vi "dllTest-ocr.vi"() -> ()   [LabVIEW 2025]
uses:
  Rectangle.ctl
  TextDecRecResult2L.ctl
panel:
  out "succ 3":i32
  out "succ 2":i32
  out "succ 5":i32
  out "deviceNum":i32
  out "succ":i32
  out "tcv":u64
  out "Image":T1(plugin-control)
  in  "PathImage":path=path "D:/Test/dllTest/images_2"
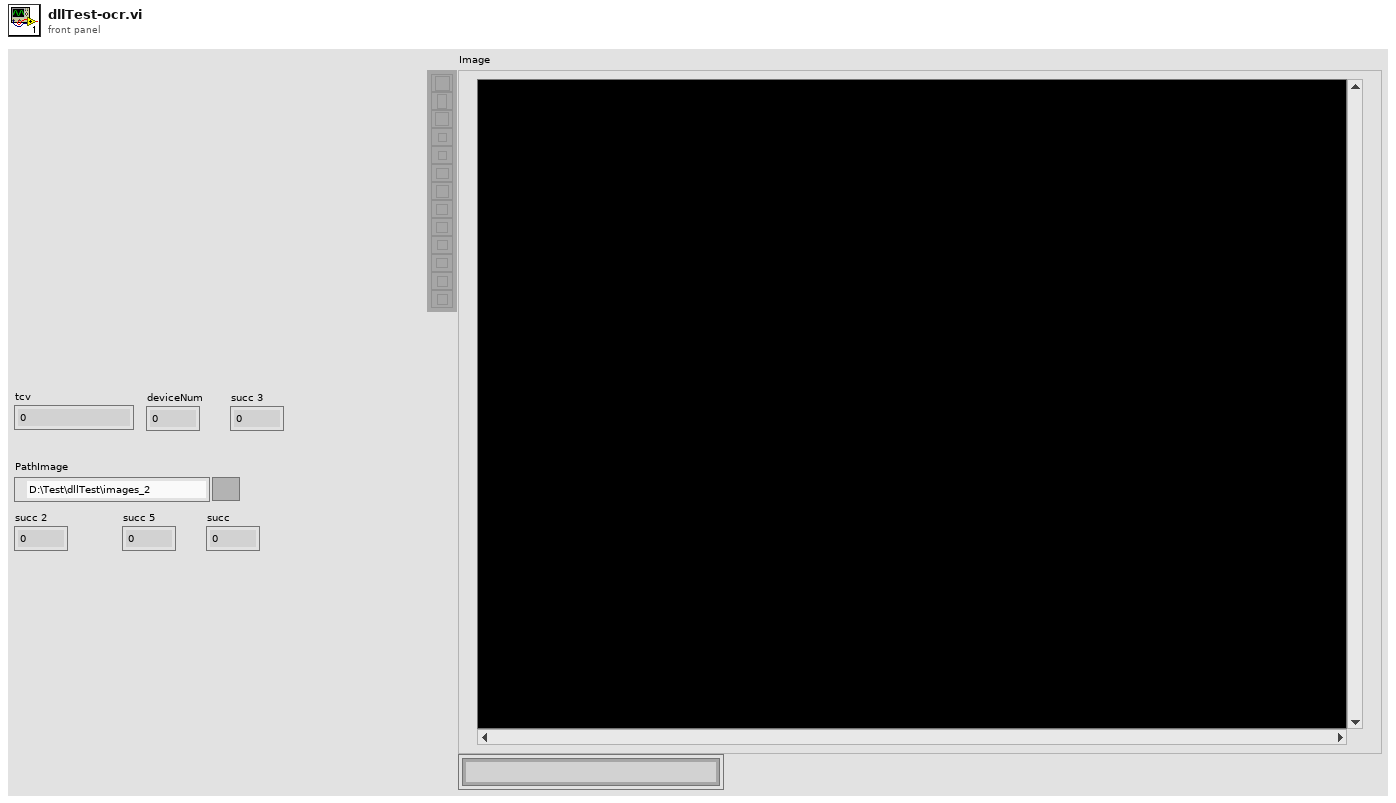
[diagram p1: front panel]
types:
  T1 = typedef "IMAQ Image.ctl" = refnum<image>
  T2 = typedef "Rectangle.ctl" = cluster{"T":i32, "L":i32, "B":i32, "R":i32}
  T3 = typedef "TextDecRecResult2L.ctl" = cluster{"imgIdx":i32, "TLx":i32, "TLy":i32, "BRx":i32, "BRy":i32, "angle":sgl, "txtLen":i32}
  T4 = cluster{"imgIdx":i32, "TLx":i32, "TLy":i32, "BRx":i32, "BRy":i32, "angle":sgl, "txtLen":i32}
  T5 = enum32{"Map Pixel Pointer", "Unmap Pixel Pointer", "Get Pixels Infos"}
  T6 = cluster{"imgIdx":i32, "TLx":i32, "TLy":i32, "BRx":i32, "BRy":i32, "angle":sgl, "txtLen":i32}[]
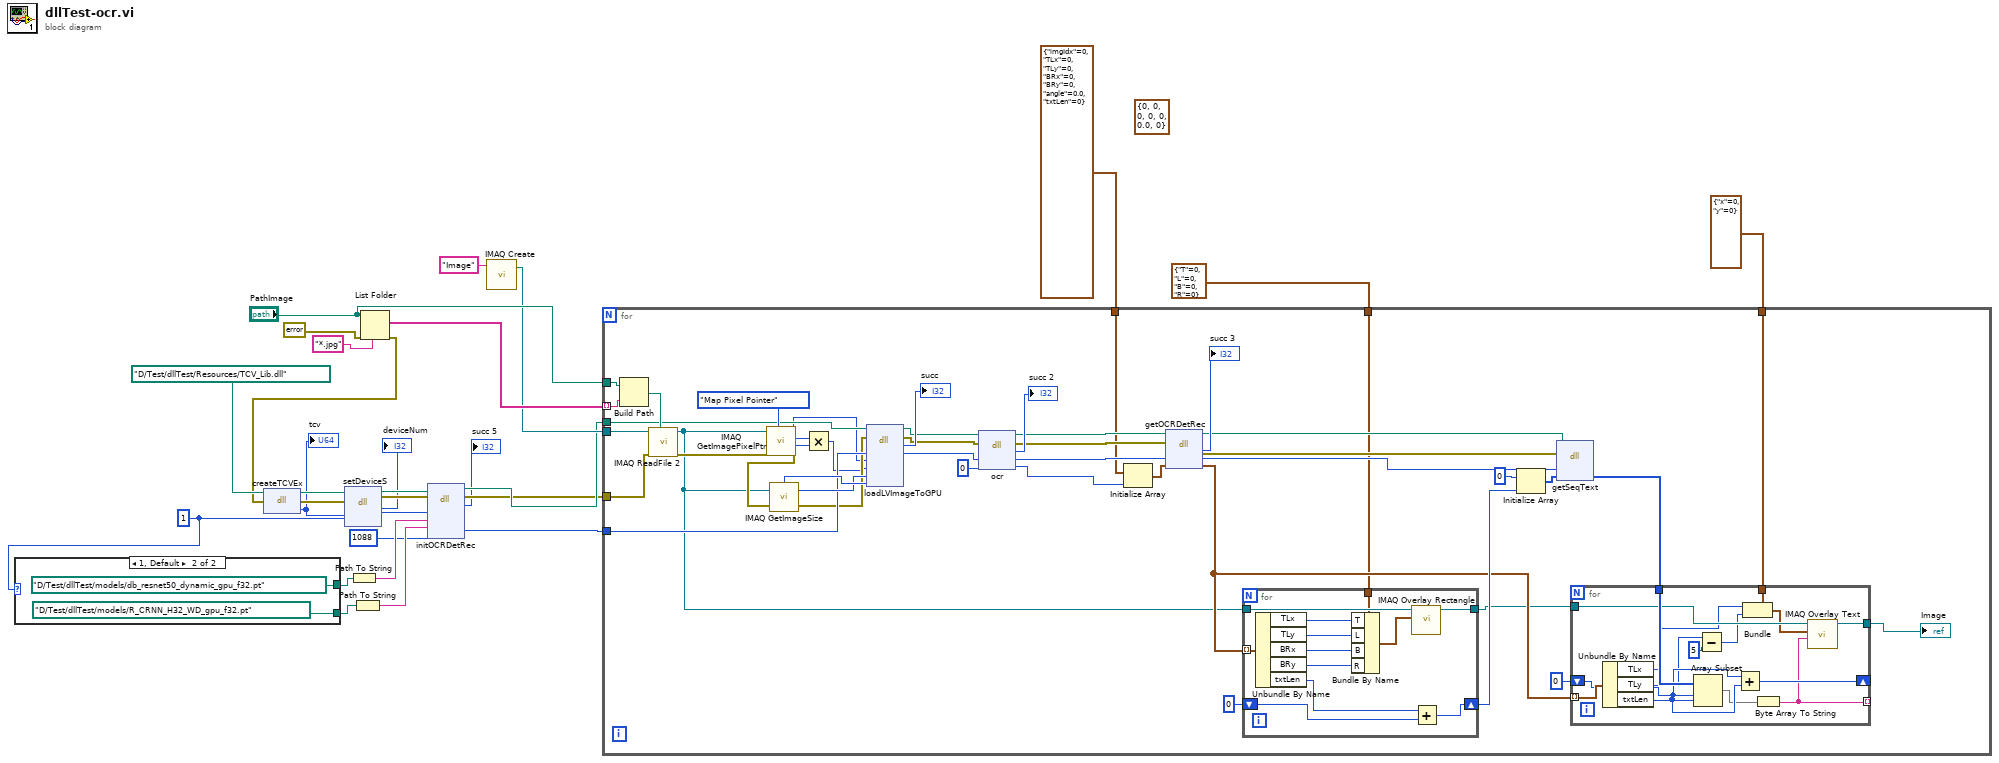
[diagram p0: block diagram]
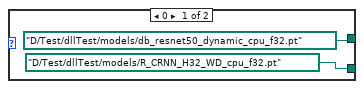
[diagram p2: hidden frame]
diagram:
  (unwired) T3 {"imgIdx"=0, "TLx"=0, "TLy"=0, "BRx"=0, "BRy"=0, "angle"=0.0, "txtLen"=0}
  w3 = 1 ("device")
  n1 = case shown="1, Default" w3 {
    tunnel: [path "D:/Test/dllTest/models/R_CRNN_H32_WD_cpu_f32.pt" ("PathModelR") path "D:/Test/dllTest/models/R_CRNN_H32_WD_gpu_f32.pt" ("PathModelR")] -> w2
    tunnel: [path "D:/Test/dllTest/models/db_resnet50_dynamic_cpu_f32.pt" ("PathModelD") path "D:/Test/dllTest/models/db_resnet50_dynamic_gpu_f32.pt" ("PathModelD")] -> w1
    frame 0 {
    }
    frame 1, Default {
    }
  }
  n2 = Path To String(path=w1) -> (string=w17:string)
  n3 = Path To String(path=w2) -> (string=w16:string)
  n4 = List Folder(path="PathImage", pattern="*.jpg", error in=errorcluster {"status"=FALSE, "code"=0, "source"=""}) -> (filenames=w26:string[], error out=w21:errorcluster)  [unwired: 1 in, 2 out]
  n5 = dll-call lib="D:/Test/dllTest/Resources/TCV_Lib.dll" fn="createTCVEx"(path in=path "D:/Test/dllTest/Resources/TCV_Lib.dll", error in=w21) -> (path out=w15:path, error out=w14:errorcluster, "tcv"=w13:u64)  [unwired: 1 in]
  "tcv" <- w13
  n6 = dll-call lib="D:/Test/dllTest/Resources/TCV_Lib.dll" fn="setDeviceS"(path in=w15, error in=w14, "TCV"=w13, "device"=w3) -> (path out=w12:path, error out=w11:errorcluster, "deviceNum"=→"deviceNum":i32, "TCV"=w10:u64)  [unwired: 2 in]
  n7 = dll-call lib="D:/Test/dllTest/Resources/TCV_Lib.dll" fn="initOCRDetRec"(path in=w12, error in=w11, "TCV"=w10, "modelPathD"=w17, "modelPathD"=w16, "targetSize"=1088) -> (path out=w20:path, error out=w19:errorcluster, "succ"=→"succ 5":i32, "TCV"=w18:u64)  [unwired: 4 in]
  n8 = call "IMAQ Create"("Image Name"="Image") -> ("New Image"=w24:T1)  [unwired: 4 in, 1 out]
  n9 = for {
    tunnel: "PathImage" -> [w77]
    tunnel: w26 -> [w76] mode=indexing
    tunnel: w24 -> [w74]
    tunnel: w18 -> [w69]
    tunnel: w20 -> [w68]
    tunnel: w19 -> [w60]
    tunnel: T4 {"imgIdx"=0, "TLx"=0, "TLy"=0, "BRx"=0, "BRy"=0, "angle"=0.0, "txtLen"=0} -> [w51]
    tunnel: T2 {"T"=0, "L"=0, "B"=0, "R"=0} -> [w37]
    tunnel: cluster{"x":i32, "y":i32} {"x"=0, "y"=0} -> [w34]
    n10 = Build Path(base path=w77, name or relative path=w76) -> (appended path=w75:path)
    n11 = call "IMAQ ReadFile 2"("File Path"=w75, "error in (no error)"=w60, "Image"=w74) -> ("error out"=w73:errorcluster, "Image Out"=w38:T1)  [unwired: 4 in, 3 out]
    n12 = call "IMAQ GetImagePixelPtr"("Function"=T5."Map Pixel Pointer", "error in (no error)"=w73, "Image"=w38) -> ("error out"=w66:errorcluster, "Pixel Size (Bytes)"=w64:i32, "LineWidth(Pixels)"=w65:i32, "Pixel Pointer out"=w62:u64)  [unwired: 3 in, 2 out]
    n13 = call "IMAQ GetImageSize"("Image"=w38, "error in (no error)"=w66) -> ("Y Resolution"=w70:i32, "X Resolution"=w71:i32, "error out"=w67:errorcluster)  [unwired: 2 in]
    n14 = Multiply(x=w65, y=w64) -> (x*y=w63:i32)
    n15 = dll-call lib="D:/Test/dllTest/Resources/TCV_Lib.dll" fn="loadLVImageToGPU"(path in=w68, error in=w67, "tcv"=w69, "imgPtr"=w62, "lw"=w63, "h"=w70, "w"=w71) -> (path out=w59:path, error out=w58:errorcluster, "succ"=→"succ":i32, "tcv"=w57:u64)  [unwired: 5 in]
    n16 = dll-call lib="D:/Test/dllTest/Resources/TCV_Lib.dll" fn="ocr"(path in=w59, error in=w58, "tcv"=w57, "totalTxt"=0) -> (path out=w54:path, error out=w53:errorcluster, "succ"=→"succ 2":i32, "tcv"=w52:u64, "totalTxt"=w50:i32)  [unwired: 1 in]
    n17 = Initialize Array(w51, w50) -> (w48:T6)
    n18 = dll-call lib="D:/Test/dllTest/Resources/TCV_Lib.dll" fn="getOCRDetRec"(path in=w54, error in=w53, "TCV"=w52, "buffer"=w48) -> (path out=w47:path, error out=w46:errorcluster, "succ"=→"succ 3":i32, "TCV"=w45:u64, "buffer"=w41:T6)  [unwired: 1 in]
    n19 = for {
      tunnel: w41 -> [w89] mode=indexing
      shift-right: [w86] -> w44
      shift-left: 0 -> [w87]
      tunnel: w38 -> [w85]
      tunnel: w37 -> [w84]
      tunnel: [w78] -> w35
      n20 = Unbundle By Name(w89) -> ("TLx"=w83:i32, "TLy"=w82:i32, "BRx"=w81:i32, "BRy"=w80:i32, "txtLen"=w88:i32)
      n21 = Bundle By Name(cluster=w84, "T"=w83, "L"=w82, "B"=w81, "R"=w80) -> (w79:T2)
      n22 = call "IMAQ Overlay Rectangle"("Rectangle"=w79, "Image"=w85) -> ("Image Out"=w78:T1)  [unwired: 8 in, 1 out]
      n23 = Add(x=w88, y=w87) -> (x+y=w86:i32)
    }
    n24 = Initialize Array "Initialize Array"(u8 0 ("element"), w44) -> (w42:u8[])
    n25 = dll-call lib="D:/Test/dllTest/Resources/TCV_Lib.dll" fn="getSeqText"(path in=w47, error in=w46, "TCV"=w45, "characters"=w42) -> ("characters"=w36:u8[])  [unwired: 3 in, 2 out]
    n26 = for {
      tunnel: w36 -> [w104]
      tunnel: w41 -> [w103] mode=indexing
      shift-right: [w101] -> _
      shift-left: 0 -> [w100]
      tunnel: [w90] -> _ mode=indexing
      tunnel: w35 -> [w98]
      tunnel: w34 -> [w97]
      tunnel: [w91] -> w33
      n27 = Unbundle By Name(w103) -> ("TLx"=w96:i32, "TLy"=w95:i32, "txtLen"=w102:i32)
      n28 = Array Subset "Array Subset"(array=w104, index=w100, length=w102) -> (w99:u8[])
      n29 = Subtract(x=w95, y=5) -> (x-y=w93:i32)
      n30 = Add(x=w100, y=w102) -> (x+y=w101:i32)
      n31 = Bundle(cluster=w97, "x"=w96, "y"=w93) -> (w92:cluster{"x":i32, "y":i32})
      n32 = Byte Array To String(unsigned byte array=w99) -> (string=w90:string)
      n33 = call "IMAQ Overlay Text"("String"=w90, "Origin"=w92, "Image"=w98) -> ("Image Out"=w91:T1)  [unwired: 7 in, 1 out]
    }
    "Image" <- w33
  }
